vi "2100_Test_Guardian Switch.vi"(0 "Semiconductor Module Context":T6, 1 "Current  Level":dbl=0.01, 2 "Master_Register_Data_Array_In":T1 {"Address" format="%.0x"}, 5 "Script_Info":T4={"Script Name"="WalkingState", "All_Scripts"=[]}, 7 "Publishable IDs":string[](array[string])=["LowPower", "Active"], 9 "USID":T3 max=15, 11 "Error In":errorcluster, 12 "Instrument_Pins":T5={"SMU_Pins"=["RF1", "RF2", "RF3", "RF4"], "HSDIO_Pins"=["CLK", "SDA"]}, 13 "Reg_Map_Bit_Name":string="RFC_SH", 14 "Reg_Map":string[][](array[string])=[["Reg Addr(0x00)", "7", "6", "5", "4", "3", "2", "1", "0"], ["0", "SPARE", "RF3_SH", "RF2_SH", "RF1_SH", "SPARE", "RF3_RFC", "RF2_RFC", "RF1_RFC"], ["1", "SPARE[7:0]", "", "", "", "", "", "", ""], ["2", "VVAR_EN", "LCM_EN", "RFC_SH", "SPARE", "VARACTOR[3:0]", "", "", ""], ["3", "SW_CTRL1_VIRTUAL[7:0]", "", "", "", "", "", "", ""], ["4", "SW_CTRL1_SWAP", "SW_CTRL1_RBSHIFT[2:0]", "", "", "SW_CTRL1_VSID[3:0]", "", "", ""], ["5", "REG_00_VIRTUAL_MASK[7:0]", "", "", "", "", "", "", ""], ["6", "LOCK_STATUS[1:0]", "", "CLK_DITHER", "FUSES_BURNED", "CLK_IDAC_CAL[3:0]", "", "", ""], ["7", "SPARE[2:0]", "", "", "ODFT_TRIM[4:0]", "", "", "", ""], ["8", "SPARE[2:0]", "", "", "HV_TRIM[4:0]", "", "", "", ""], ["9", "TEST_MUX[2:0]", "", "", "SPARE[1:0]", "", "MEMS_BG_TC[1:0]", "", "MEMSCP_RCM"], ["A", "CP_BOOST_OVRD_EN", "SPARE[2:0]", "", "", "PS_OFF_TIMER[1:0]", "", "PS_ON_TIMER[1:0]", ""], ["0", "", "", "", "", "", "", "", ""], ["D", "Reserved[1:0]", "", "WD_HI_EVENT_CNT[5:0]", "", "", "", "", ""], ["E", "VERSION_ID[7:0]", "", "", "", "", "", "", ""], ["F", "Reserved", "COUNT_200_LSB[6:0]", "", "", "", "", "", ""], ["10", "CLK_DIV2_EN", "Spare", "ODFT_EN", "HV_HYST[4:0]", "", "", "", ""], ["0", "", "", "", "", "", "", "", ""], ["12", "SHORT_FUSE", "FUSE_BURN", "STROBE_EN", "VIO_OK", "RTH[1:0]", "", "FUSE_LOAD_MAN_EN", "FUSE_LOAD"], ["13", "RR_ACK_EN", "Reserved", "ACK_POSITION[1:0]", "", "SuBUS_DRIVE_STRENGTH[3:0]", "", "", ""], ["14", "TM_IO_EN", "TM_IO_SEL", "SuBUS_OVS[1:0]", "", "Reserved[3:0]", "", "", ""], ["15", "Reserved[4:0]", "", "", "", "", "SuBUS_VERSION_PRESENT", "SuBUS_VOLTAGE", "SuBUS_FLAVOR_DEF"], ["16", "PROG_STROBE1_DUR[7:0]", "", "", "", "", "", "", ""], ["17", "PROG_STROBE0_DUR[7:0]", "", "", "", "", "", "", ""], ["18", "Reserved[2:0]", "", "", "EFUSE_SINGLE_ADDR_SEL[4:0]", "", "", "", ""], ["19", "POLL_ADR[4:0]", "", "", "", "", "POLL_BC[2:0]", "", ""], ["1A", "SOFTWARE_RESET", "Reserved[6:0]", "", "", "", "", "", ""], ["1B", "Reserved[7:0]", "", "", "", "", "", "", ""], ["1C", "PWR_MODE_1", "PWR_MODE_0", "TRIGGER_MASK[2:0]", "", "", "TRIGGER[2:0]", "", ""], ["1D", "PRODUCT_ID[7:0]", "", "", "", "", "", "", ""], ["1E", "MANUFACTURER_ID_LSB[7:0]", "", "", "", "", "", "", ""], ["1F", "MANUFACTURER_ID_MSB[3:0]", "", "", "", "USID[3:0]", "", "", ""]]) -> (6 "Master_Register_Data_Array_Out":T1 {"Address" format="%.0x"}, 8 "R_Guardian":dbl[](array[numeric]) format="%#_6p", 15 "Error Out":errorcluster)   [LabVIEW 2013]
uses:
  Controls/USID.ctl
  <vilib>/NI_TestStand_SemiconductorModule/NI_TestStand_Semiconductor_Module.lvlibp/PinMap/General/SemiconductorModuleContext.ctl
  Controls/Master_Reg_Data_Array.ctl
  Controls/Reg_Address_Data.ctl
  <vilib>/NI_TestStand_SemiconductorModule/NI_TestStand_Semiconductor_Module.lvlibp/PinMap/General/Publish/PublishDataDoubleFunctionalTest.vi
  <vilib>/NI_TestStand_SemiconductorModule/NI_TestStand_Semiconductor_Module.lvlibp
panel:
  out "R Array":dbl[][](array[numeric]) format="%#_6p"
  in  "Tab Control":enum32{"Test Info", "Instrument Settings"}(tab)
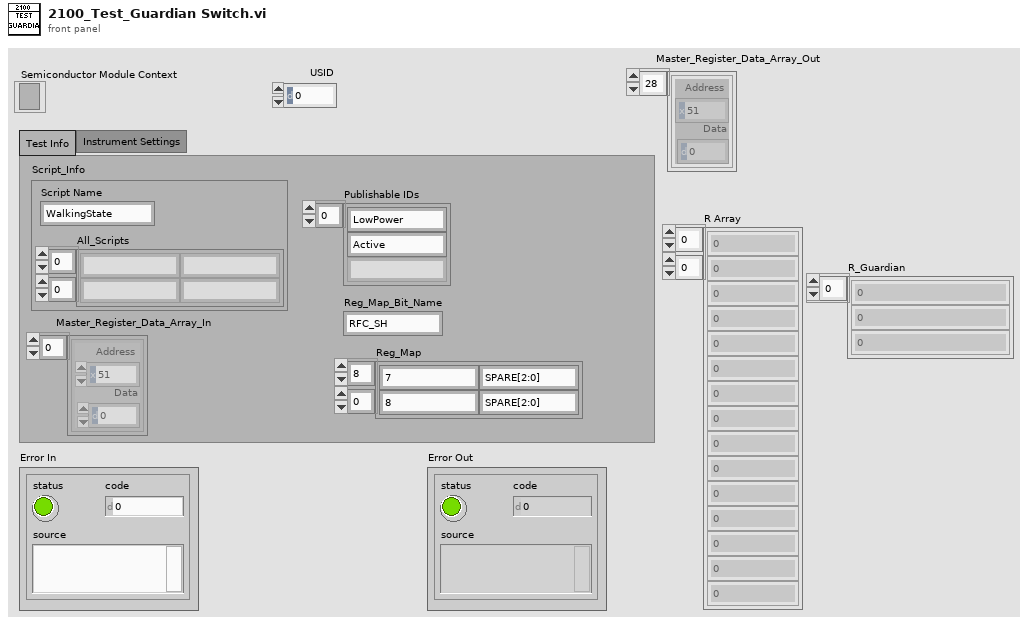
[diagram p1: front panel]
types:
  T1 = typedef "Master_Reg_Data_Array.ctl" = T2[]
  T2 = typedef "Reg_Address_Data.ctl" = cluster{"Address":u8, "Data":u8}
  T3 = typedef "USID.ctl" = u8
  T4 = cluster{"Script Name":string, "All_Scripts":string[][]}
  T5 = cluster{"SMU_Pins":string[], "HSDIO_Pins":string[]}
  T6 = typedef "NI_TestStand_Semiconductor_Module.lvlibp/SemiconductorModuleContext.ctl" = refnum<k7>
  T7 = typedef "Script Functions_Array.ctl" = enum16{"Reg_Write", "Bit_Write", "Delay", "Read", "Measure"}[]
  T8 = enum16{"Reg_Write", "Bit_Write", "Delay", "Read", "Measure"}
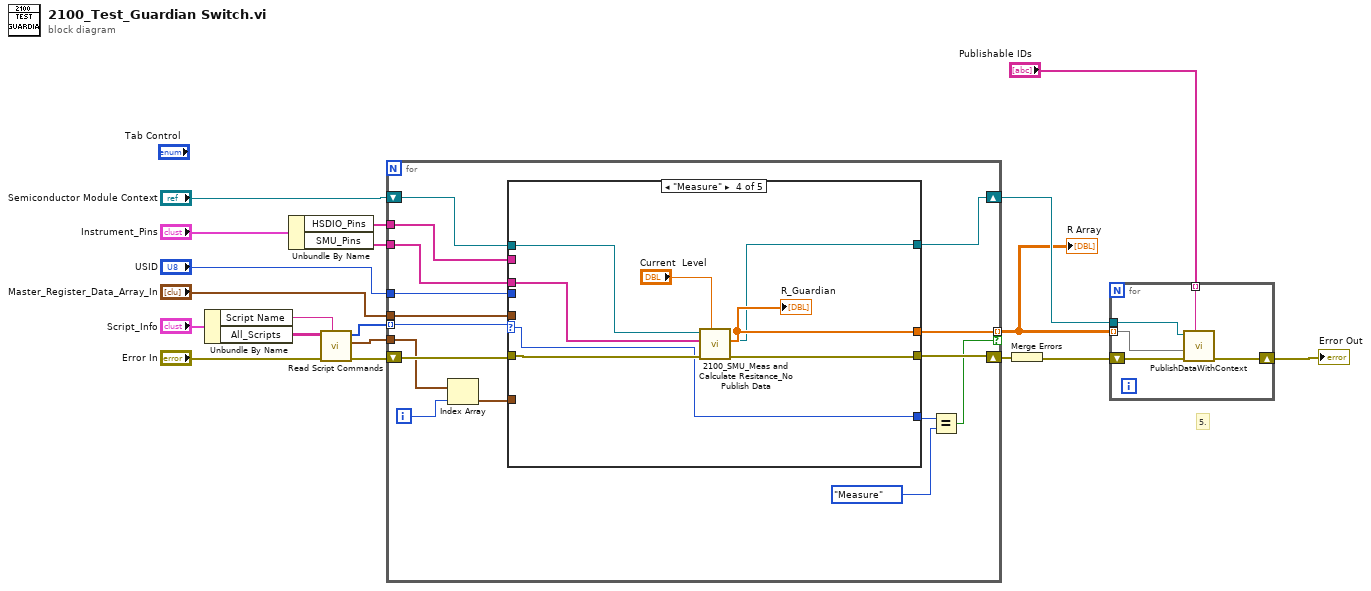
[diagram p0: block diagram]
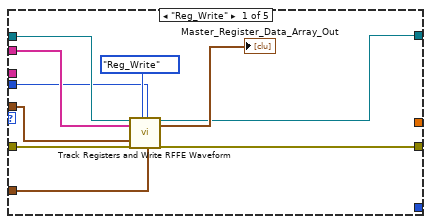
[diagram p2: hidden frame]
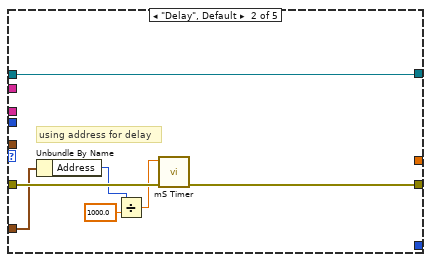
[diagram p3: hidden frame]
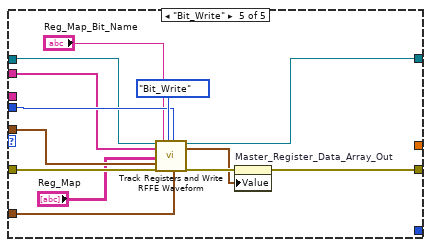
[diagram p5: hidden frame]
diagram:
  # "5."
  n1 = Unbundle By Name("Script_Info") -> ("Script Name"=w7:string, "All_Scripts"=w8:string[][])
  n2 = Unbundle By Name("Instrument_Pins") -> ("HSDIO_Pins"=w11:string[], "SMU_Pins"=w10:string[])
  n3 = call "Read Script Commands.vi"("Test Name"=w7, "Error In"="Error In", "All_Scripts"=w8) -> ("Error Out"=w16:errorcluster, "Script_Data"=w17:T2[], "Script_Functions"=w18:T7)  [unwired: 5 in, 1 out]
  n4 = for {
    tunnel: "USID" -> [w30]
    tunnel: w18 -> [w29] mode=indexing
    tunnel: w17 -> [w33]
    tunnel: w11 -> [w34]
    shift-right: [w27] -> w14
    shift-left: w16 -> [w35]
    tunnel: "Master_Register_Data_Array_In" -> [w31]
    tunnel: w10 -> [w26]
    tunnel: [w25] -> w3 mode=indexing if=w21
    shift-right: [w24] -> w4
    shift-left: "Semiconductor Module Context" -> [w20]
    i -> [w28]
    n5 = Index Array(array=w33, index=w28) -> (element=w32:T2)
    n6 = case shown="\"Measure\"" w29 {
      selector: w29 -> [_ _ _ w55 _]
      tunnel: w32 -> [w40 w51 _ _ w68]
      tunnel: w35 -> [w45 w52 w54 w60 w75]
      tunnel: w30 -> [w37 _ _ _ w73]
      tunnel: w20 -> [w43 w46 w53 w58 w72]
      tunnel: w34 -> [w42 _ _ _ w71]
      tunnel: [w44 w50 w54 w61 w65] -> w27
      tunnel: w31 -> [w39 _ _ _ w69]
      tunnel: w26 -> [_ _ _ w62 _]
      tunnel: [_ _ _ w57 _] -> w25
      tunnel: [w36 w46 w53 w56 w63] -> w24
      tunnel: [_ _ _ w55 _] -> w23
      frame "Reg_Write" {
        n7 = call "Track Registers and Write RFFE Waveform.vi"("Semiconductor Module Context"=w43, "Pins"=w42, "Master_Register_Data_Array_In"=w39, "Error In"=w45, "Script_Functions"=enum16{"Reg_Write", "Bit_Write"}."Reg_Write", "USID"=w37, "Reg_Address_Data"=w40) -> ("Semiconductor Module Context Out"=w36:T6, "Master_Register_Data_Array_Out"=→"Master_Register_Data_Array_Out":T1, "Error Out"=w44:errorcluster)  [unwired: 10 in]
      }
      frame "Delay", Default {
        # "using address for delay"
        n8 = Unbundle By Name(w51) -> ("Address"=w48:u8)
        n9 = Divide(x=w48, y=1000.0) -> (x/y=w47:dbl)
        n10 = call "mS Timer.vi"("Error In"=w52, "Delay(S)"=w47) -> ("Error Out"=w50:errorcluster)  [unwired: 9 in]
      }
      frame "Read" {
      }
      frame "Measure" {
        n11 = call "2100_SMU_Meas and Calculate Resitance_No Publish Data.vi"("Current  Level"="Current  Level", "error in (no error)"=w60, "Pins"=w62, "Semiconductor Module Context"=w58) -> ("error Out"=w61:errorcluster, "R Array"=w57:dbl[], "Semiconductor Module Context Out"=w56:T6)  [unwired: 5 in]
        "R_Guardian" <- w57
      }
      frame "Bit_Write" {
        n12 = call "Track Registers and Write RFFE Waveform.vi"("Semiconductor Module Context"=w72, "Pins"=w71, "Reg_Map"="Reg_Map", "Master_Register_Data_Array_In"=w69, "Error In"=w75, "Reg_Map_Bit_Name"="Reg_Map_Bit_Name", "Script_Functions"=enum16{"Reg_Write", "Bit_Write"}."Bit_Write", "USID"=w73, "Reg_Address_Data"=w68) -> ("Semiconductor Module Context Out"=w63:T6, "Master_Register_Data_Array_Out"=w64:T1, "Error Out"=w66:errorcluster)  [unwired: 8 in]
        n13 = property on="Master_Register_Data_Array_Out" class="Arr (strict)"(error in=w66, "Value"=w64) -> (error out=w65:errorcluster)  [unwired: 1 in, 1 out]
      }
    }
    n14 = Equal?(x=w23, y=T8."Measure" ("Enum")) -> (x = y?=w21:bool)
  }
  "R Array" <- w3
  n15 = Merge Errors(w14) -> (w6:errorcluster)
  n16 = for {
    shift-right: [w80] -> w5
    shift-left: w6 -> [w79]
    tunnel: w3 -> [w76] mode=indexing
    tunnel: w4 -> [w78]
    tunnel: "Publishable IDs" -> [w77] mode=indexing
    n17 = call-poly <vilib>:"PublishDataWithContext.vi"("Published Data Id"=w77, "error in (no error)"=w79, "Data In"=w76, "Semiconductor Module Context"=w78) -> ("error out"=w80:errorcluster)  [unwired: 6 in, 1 out]
  }
  "Error Out" <- w5
